vi "Send Message to Colleague.vi"(8 "error in (no error)":errorcluster caption="错误输入（无错误）", 10 "Message.lvclass":refnum<class "Message.lvclass">, 11 "中介者（抽象） 输入":refnum<class "Mediator.lvclass"> caption="DNL_LabVIEW Object in") -> (0 "error out":errorcluster caption="错误输出", 3 "中介者（抽象） 输出":refnum<class "Mediator.lvclass"> caption="DNL_LabVIEW Object out")   [LabVIEW 2011, in "Mediator.lvclass"]
uses:
  Mediator.lvclass
  Mediator.lvclass/Mediator.ctl
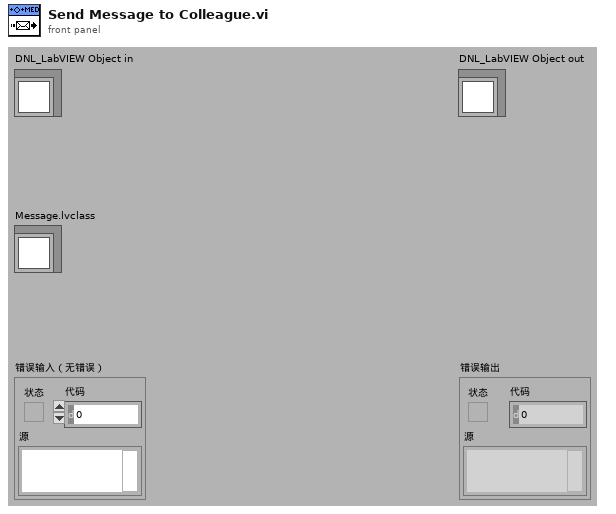
[diagram p1: front panel]
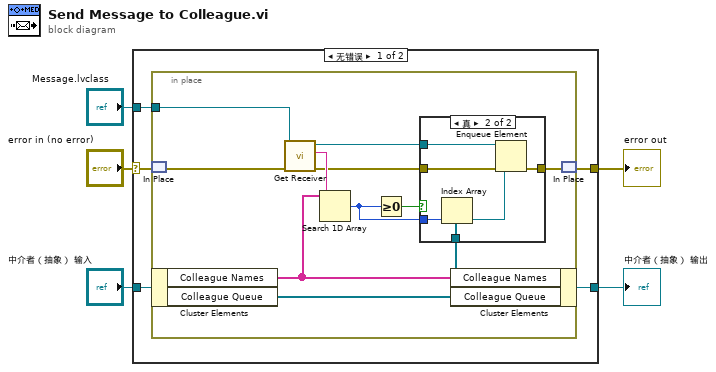
[diagram p0: block diagram]
diagram:
  n1 = case shown="无错误" "error in (no error)" {
    selector: "error in (no error)" -> [w8 w29]
    tunnel: [w7 w29] -> w4
    tunnel: [w6 w28] -> w2
    tunnel: "中介者（抽象） 输入" -> [w10 w28]
    tunnel: "Message.lvclass" -> [w9 _]
    frame No Error {
      n2 = in-place {
        in-place-border: w9 -> [w19]
        n3 = in-place-match #1(w8) -> (w15:errorcluster)
        n4 = in-place-cluster #2(w10) -> ("Colleague Names"=w12:string[], "Colleague Queue"=w11:refnum<queue>[])
        n5 = call "Get Receiver.vi"("error in (no error)"=w15, "Message输入"=w19) -> ("error out"=w14:errorcluster, "Receiver"=w20:string, "Message输出"=w16:refnum<class "Message.lvclass">)  [unwired: 7 in]
        n6 = Search 1D Array(1D array=w12, element=w20) -> (index of element=w17:i32)  [unwired: 1 in]
        n7 = Greater Or Equal To 0?(x=w17) -> (x >= 0?=w18:bool)
        n8 = case shown="真" w18 {
          tunnel: w11 -> [_ w27]
          tunnel: w17 -> [_ w26]
          tunnel: w16 -> [_ w24]
          tunnel: w14 -> [w21 w23]
          tunnel: [w21 w22] -> w13
          frame False {
          }
          frame True {
            n9 = Index Array(array=w27, index=w26) -> (element=w25:refnum<queue>)
            n10 = Enqueue Element(queue=w25, element=w24, error in (no error)=w23) -> (error out=w22:errorcluster)  [unwired: 1 in, 2 out]
          }
        }
        n11 = in-place-cluster #2("Colleague Names"=w12, "Colleague Queue"=w11) -> (w6:refnum<class "Mediator.lvclass">)
        n12 = in-place-match #1(w13) -> (w7:errorcluster)
      }
    }
    frame Error {
    }
  }
  "error out" <- w4
  "中介者（抽象） 输出" <- w2
